vi "from_data_and_type_descriptor.vi"(5 "LVData in":refnum<class "variant.lvclass">, 8 "error in (no error)":errorcluster, 10 "data":refnum<class "Bytes.lvclass">, 11 "type_descriptor":refnum<class "Bytes.lvclass">) -> (0 "error out":errorcluster, 3 "LVData out":refnum<class "variant.lvclass">)   [LabVIEW 2020, in "variant.lvlib" / "variant.lvclass"]
uses:
  variant.lvclass
  Bytes/Bytes.lvclass
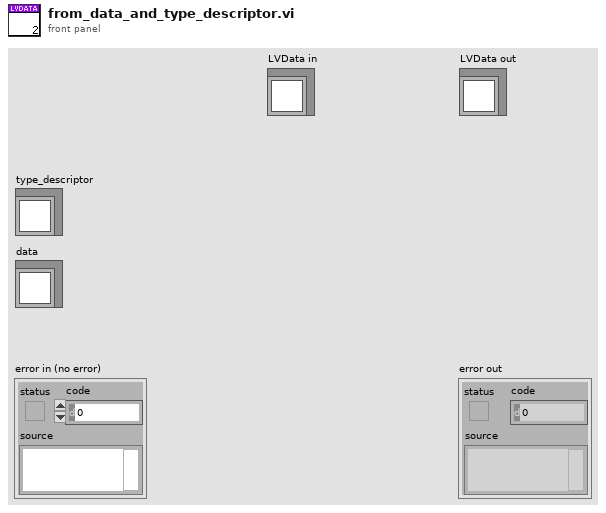
[diagram p1: front panel]
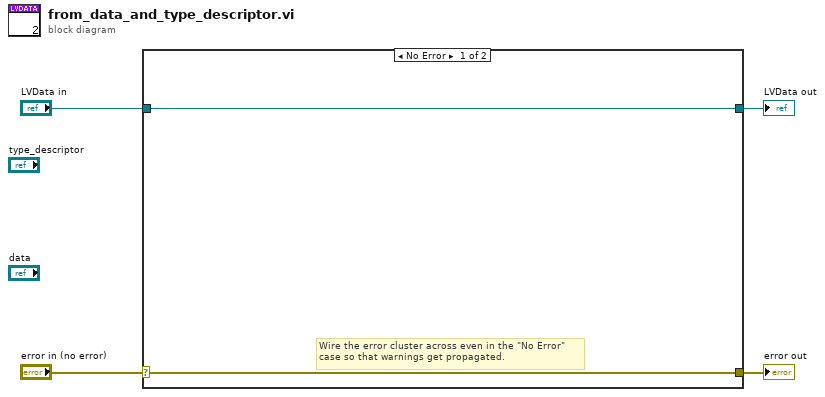
[diagram p0: block diagram]
diagram:
  n1 = case shown="No Error" "error in (no error)" {
    selector: "error in (no error)" -> [w5 w8]
    tunnel: [w5 w8] -> w3
    tunnel: [w6 w7] -> w1
    tunnel: "LVData in" -> [w6 w7]
    frame No Error {
      # "Wire the error cluster across even in the \"No Error\"\ncase so that warnings get propagated."
    }
    frame Error {
    }
  }
  "error out" <- w3
  "LVData out" <- w1
